vi "LibXML_GetNodeAttributeNamed.vi"(8 "error in":errorcluster, 10 "attribute name":string, 11 "node":u32) -> (0 "error out":errorcluster, 3 "string pointer":u32)   [LabVIEW 2019, in "Tools.lvlib" / "LibXML.lvlib"]
doc: "Gets the string pointer to an attribute (by name input) at the node input."
uses:
  LibXML.lvlib
  dll/lXMLwrap.dll
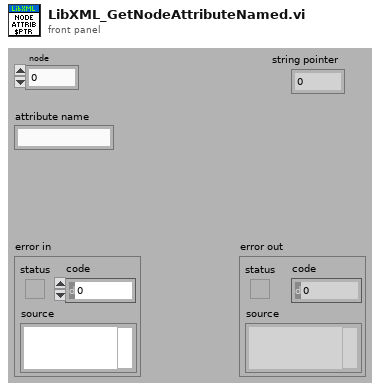
[diagram p1: front panel]
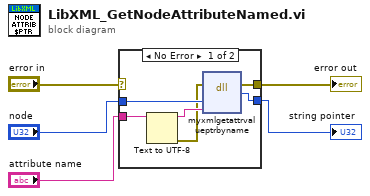
[diagram p0: block diagram]
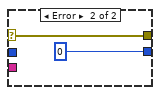
[diagram p2: hidden frame]
diagram:
  n1 = case shown="No Error" "error in" {
    selector: "error in" -> [_ w13]
    tunnel: [w10 w13] -> w4
    tunnel: [w11 u32 0 ("return type")] -> w3
    tunnel: "node" -> [w9 _]
    tunnel: "attribute name" -> [w8 _]
    frame No Error {
      n2 = Text to UTF-8(11:w8) -> (0:w6:errorcluster, 3:w7:string)  [unwired: 2 in]
      n3 = dll-call lib="C:/Projects/_Prywatne/MyCIT/Framework/Tools/XML/LibXML/dll/lXMLwrap.dll" fn="myxmlgetattrvalueptrbyname"(error in=w6, "node"=w9, "attribte_name"=w7) -> (error out=w10:errorcluster, "return type"=w11:u32)  [unwired: 4 in, 1 out]
    }
    frame Error {
    }
  }
  "error out" <- w4
  "string pointer" <- w3
